vi "ClassBannerEditor_SetText.vi"(4 "error in (no error)":errorcluster, 5 "Value":string, 6 "Container State":T4, 7 "Display State In":T1={"CurrentIcon"={"Icon Text"="Default", "RectangleColors"={"Border"=0, "Background"=16448250}, "FontSettings"={"Size"=8, "Capitalize text"=TRUE, "TextColor"=0}}}) -> (0 "error out":errorcluster, 3 "Display State Out":T1={"CurrentIcon"={"Icon Text"="Default", "RectangleColors"={"Border"=0, "Background"=16448250}, "FontSettings"={"Size"=8, "Capitalize text"=TRUE, "TextColor"=0}}})   [LabVIEW 2014, in "ClassBannerEditor.xctl"]
uses:
  ClassBannerEditor.xctl
  <vilib>/_xctls/Container State.ctl
  ClassBannerEditor_State.ctl
  <vilib>/LabVIEW Icon API/API_Rectangle Colors.ctl
  ClassBannerEditor_FontSettings.ctl
  <vilib>/_xctls/XControlSupport.lvlib
  <vilib>/LabVIEW Icon API/LabVIEW Icon API.lvlib
panel:
  # "Replace the Value Control below with a Control of desired type.\nDo not remove this Control or the others from the connector pane.\nDo not change the connector pane pattern.\nThe Value control should always be the third terminal from top on the input side in the connector pane."
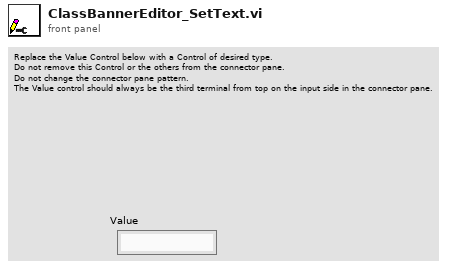
[diagram p1: front panel]
types:
  T1 = typedef "ClassBannerEditor.xctl/ClassBannerEditor_State.ctl" = cluster{"CurrentIcon":cluster{"Icon Text":string, "RectangleColors":T2, "FontSettings":T3}}
  T2 = typedef "LabVIEW Icon API.lvlib/API_Rectangle Colors.ctl" = cluster{"Border":u32, "Background":u32}
  T3 = typedef "ClassBannerEditor.xctl/ClassBannerEditor_FontSettings.ctl" = cluster{"Size":u8, "Capitalize text":bool, "TextColor":u32}
  T4 = typedef "XControlSupport.lvlib/Container State.ctl" = cluster{"Indicator?":bool, "Run Mode?":bool, " Refnum":refnum<vi>}
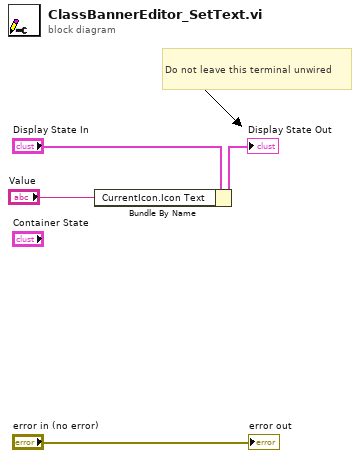
[diagram p0: block diagram]
diagram:
  # "Do not leave this terminal unwired"
  n1 = Bundle By Name(cluster="Display State In", "CurrentIcon.Icon Text"="Value") -> (→"Display State Out":T1)
  "error out" <- "error in (no error)"
